vi "scecmd-list-to-json.vi"(11 "sce-cmd-list":cluster{"字符串":string, "数组 2":string[]}[](array[cluster])) -> (0 "LV Text":string, 3 "<JSON>":string caption="<JSON>Object")   [LabVIEW 2019]
uses:
  b78e4e2b-07cc-4402-99e5-c8c8689a2c4a.vi
  79eddf31-7dbf-49f6-a314-521278fd7013.vi
  3a01fc26-5e33-4aa7-adf9-b5ac6e867385.vi
  10d2d137-27d5-4f8a-8f99-ee01ed841b88.vi
  6bf9a7dc-aad9-4d5c-b2fa-1059882cb968.vi
  <vilib>/JDP Science/JSONtext/support/Format JSON Object.vi
  <vilib>/JDP Science/JSONtext/Variant to JSON Text.vi
  <vilib>/JDP Science/JSONtext/Get all Object Items.vi
  <vilib>/JDP Science/JSONtext/Set Multiple Object Items.vi
  <vilib>/JDP Science/JSONtext/JSONtext.lvlib
  <vilib>/addons/Tools/Unicode/UTF8 Tools.lvlib
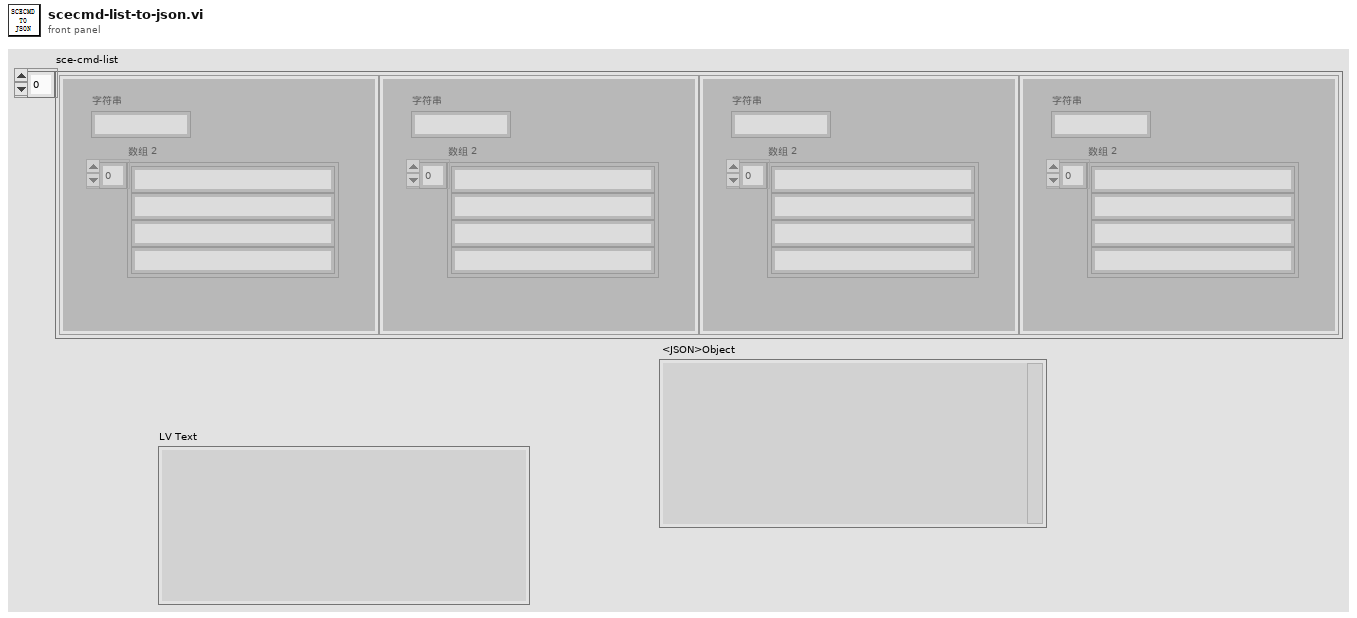
[diagram p1: front panel]
types:
  T1 = cluster{"场景":string, "open":cluster{"ID":dbl, "payload":string[]}, "close":cluster{"ID":dbl, "payload":string[]}, "common":cluster{"ID":dbl, "payload":string[]}}[]
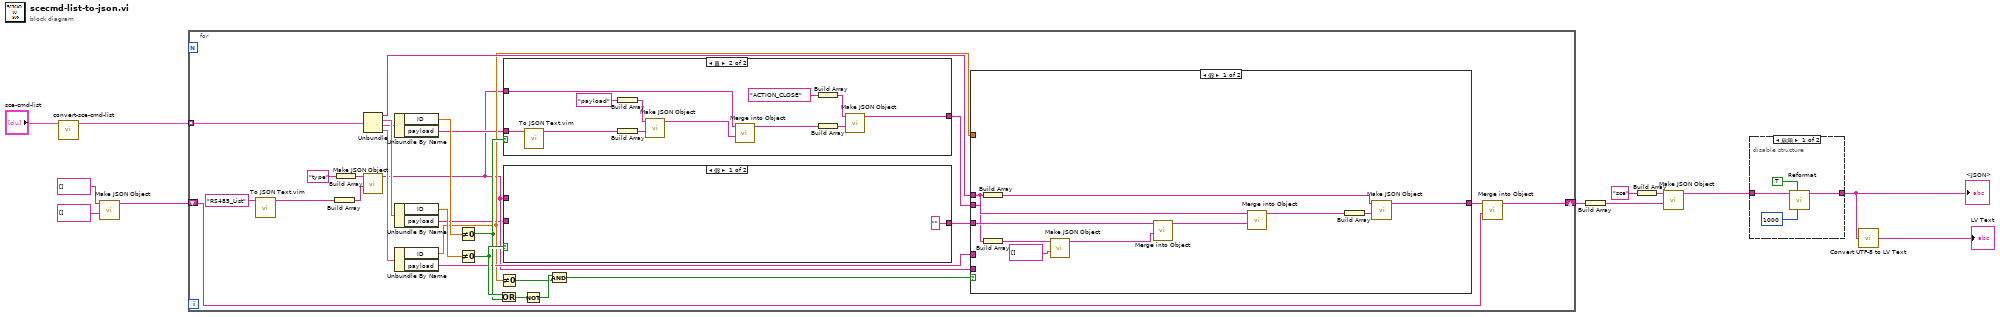
[diagram p0: block diagram]
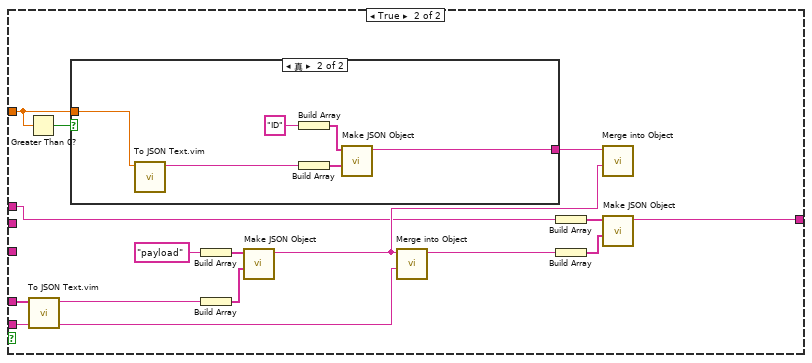
[diagram p3: hidden frame]
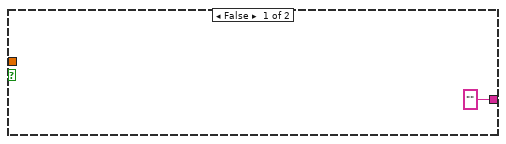
[diagram p4: hidden frame]
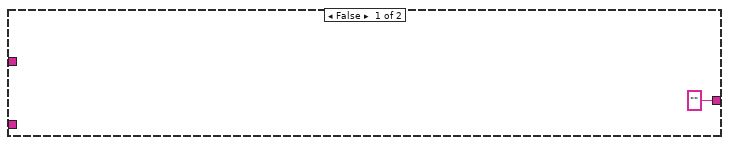
[diagram p5: hidden frame]
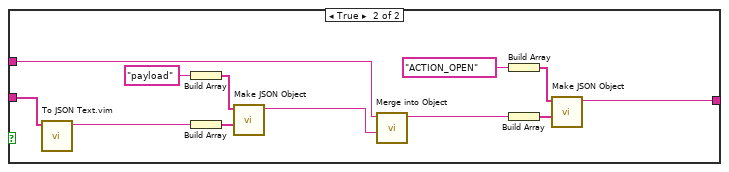
[diagram p6: hidden frame]
diagram:
  n1 = call "convert-sce-cmd-list.vi"("sce-cmd-list"="sce-cmd-list") -> ("场景-cmd-list"=w11:T1)  [unwired: 10 in]
  n2 = call <vilib>:"Make JSON Object.vi"("JSON Items"=string[] [], "Item Names"=string[] []) -> ("<JSON>"=w8:string)  [unwired: 8 in, 1 out]
  n3 = for {
    tunnel: w11 -> [w40] mode=indexing
    shift-right: [w14] -> w6
    shift-left: w8 -> [w13]
    n4 = call "To JSON Text.vim"("Anything"="RS485_List") -> ("<JSON>"=w26:string)  [unwired: 9 in, 1 out]
    n5 = Build Array(w26) -> (w25:string[])
    n6 = Build Array("type") -> (w27:string[])
    n7 = Unbundle(w40) -> ("场景"=w23:string, "open"=w39:cluster{"ID":dbl, "payload":string[]}, "close"=w38:cluster{"ID":dbl, "payload":string[]}, "common"=w37:cluster{"ID":dbl, "payload":string[]})
    n8 = call <vilib>:"Make JSON Object.vi"("JSON Items"=w25, "Item Names"=w27) -> ("<JSON>"=w19:string)  [unwired: 8 in, 1 out]
    n9 = Unbundle By Name(w38) -> ("ID"=w35:dbl, "payload"=w20:string[])
    n10 = Unbundle By Name(w39) -> ("ID"=w36:dbl, "payload"=w18:string[])
    n11 = Unbundle By Name(w37) -> ("ID"=w21:dbl, "payload"=w22:string[])
    n12 = Not Equal To 0?(x=w35) -> (x != 0?=w33:bool)
    n13 = Not Equal To 0?(x=w36) -> (x != 0?=w34:bool)
    n14 = Not Equal To 0?(x=w21) -> (x != 0?=w30:bool)
    n15 = Or(x=w34, y=w33) -> (x .or. y?=w32:bool)
    n16 = case shown="真" w33 {
      tunnel: w20 -> [_ w84]
      tunnel: w19 -> [_ w81]
      tunnel: ["" ("<JSON>") w75] -> w17
      frame False {
      }
      frame True {
        n17 = call "To JSON Text.vim"("Anything"=w84) -> ("<JSON>"=w83:string)  [unwired: 9 in, 1 out]
        n18 = Build Array("payload") -> (w85:string[])
        n19 = Build Array(w83) -> (w82:string[])
        n20 = call <vilib>:"Make JSON Object.vi"("JSON Items"=w82, "Item Names"=w85) -> ("<JSON>"=w80:string)  [unwired: 8 in, 1 out]
        n21 = call <vilib>:"Merge into Object.vi"("JSON Object to Merge"=w80, "JSON"=w81) -> ("<JSON>"=w76:string)  [unwired: 7 in, 1 out]
        n22 = Build Array("ACTION_CLOSE") -> (w79:string[])
        n23 = Build Array(w76) -> (w78:string[])
        n24 = call <vilib>:"Make JSON Object.vi"("JSON Items"=w78, "Item Names"=w79) -> ("<JSON>"=w75:string)  [unwired: 8 in, 1 out]
      }
    }
    n25 = case shown="假" w34 {
      tunnel: w19 -> [_ w94]
      tunnel: w18 -> [_ w93]
      tunnel: ["" ("<JSON>") w88] -> w16
      frame False {
      }
      frame True {
        n26 = call "To JSON Text.vim"("Anything"=w93) -> ("<JSON>"=w97:string)  [unwired: 9 in, 1 out]
        n27 = Build Array("payload") -> (w96:string[])
        n28 = Build Array(w97) -> (w98:string[])
        n29 = call <vilib>:"Make JSON Object.vi"("JSON Items"=w98, "Item Names"=w96) -> ("<JSON>"=w99:string)  [unwired: 8 in, 1 out]
        n30 = call <vilib>:"Merge into Object.vi"("JSON Object to Merge"=w99, "JSON"=w94) -> ("<JSON>"=w91:string)  [unwired: 7 in, 1 out]
        n31 = Build Array("ACTION_OPEN") -> (w89:string[])
        n32 = Build Array(w91) -> (w90:string[])
        n33 = call <vilib>:"Make JSON Object.vi"("JSON Items"=w90, "Item Names"=w89) -> ("<JSON>"=w88:string)  [unwired: 8 in, 1 out]
      }
    }
    n34 = Not(x=w32) -> (.not. x?=w31:bool)
    n35 = And(x=w31, y=w30) -> (x .and. y?=w29:bool)
    n36 = case shown="假" w29 {
      tunnel: w23 -> [w45 w56]
      tunnel: w22 -> [_ w59]
      tunnel: w21 -> [_ w66]
      tunnel: w19 -> [_ w57]
      tunnel: w17 -> [w48 _]
      tunnel: w16 -> [w50 _]
      tunnel: [w41 w52] -> w15
      frame False {
        n37 = Build Array(w45) -> (w44:string[])
        n38 = Build Array(w45) -> (w51:string[])
        n39 = call <vilib>:"Make JSON Object.vi"("JSON Items"=string[] [], "Item Names"=w51) -> ("<JSON>"=w49:string)  [unwired: 8 in, 1 out]
        n40 = call <vilib>:"Merge into Object.vi"("JSON Object to Merge"=w49, "JSON"=w50) -> ("<JSON>"=w47:string)  [unwired: 7 in, 1 out]
        n41 = call <vilib>:"Merge into Object.vi"("JSON Object to Merge"=w47, "JSON"=w48) -> ("<JSON>"=w43:string)  [unwired: 7 in, 1 out]
        n42 = Build Array(w43) -> (w42:string[])
        n43 = call <vilib>:"Make JSON Object.vi"("JSON Items"=w42, "Item Names"=w44) -> ("<JSON>"=w41:string)  [unwired: 8 in, 1 out]
      }
      frame True {
        n44 = Greater Than 0?(x=w66) -> (x > 0?=w65:bool)
        n45 = call "To JSON Text.vim"("Anything"=w59) -> ("<JSON>"=w62:string)  [unwired: 9 in, 1 out]
        n46 = case shown="真" w65 {
          tunnel: w66 -> [_ w69]
          tunnel: ["" ("<JSON>") w68] -> w60
          frame False {
          }
          frame True {
            n47 = call "To JSON Text.vim"("Anything"=w69) -> ("<JSON>"=w72:string)  [unwired: 9 in, 1 out]
            n48 = Build Array("ID") -> (w71:string[])
            n49 = Build Array(w72) -> (w73:string[])
            n50 = call <vilib>:"Make JSON Object.vi"("JSON Items"=w73, "Item Names"=w71) -> ("<JSON>"=w68:string)  [unwired: 8 in, 1 out]
          }
        }
        n51 = Build Array("payload") -> (w63:string[])
        n52 = Build Array(w62) -> (w61:string[])
        n53 = call <vilib>:"Make JSON Object.vi"("JSON Items"=w61, "Item Names"=w63) -> ("<JSON>"=w58:string)  [unwired: 8 in, 1 out]
        n54 = call <vilib>:"Merge into Object.vi"("JSON Object to Merge"=w57, "JSON"=w58) -> ("<JSON>"=w54:string)  [unwired: 7 in, 1 out]
        n55 = Build Array(w56) -> (w55:string[])
        n56 = Build Array(w54) -> (w53:string[])
        n57 = call <vilib>:"Merge into Object.vi"("JSON Object to Merge"=w58, "JSON"=w60) -> ()  [unwired: 7 in, 2 out]
        n58 = call <vilib>:"Make JSON Object.vi"("JSON Items"=w53, "Item Names"=w55) -> ("<JSON>"=w52:string)  [unwired: 8 in, 1 out]
      }
    }
    n59 = call <vilib>:"Merge into Object.vi"("JSON Object to Merge"=w13, "JSON"=w15) -> ("<JSON>"=w14:string)  [unwired: 7 in, 1 out]
  }
  n60 = Build Array(w6) -> (w5:string[])
  n61 = Build Array("sce") -> (w4:string[])
  n62 = call <vilib>:"Make JSON Object.vi"("JSON Items"=w5, "Item Names"=w4) -> ("<JSON>"=w2:string)  [unwired: 8 in, 1 out]
  n63 = disable-structure shown="启用" {
    disable-tunnel: w2 -> [w103 w104]
    disable-tunnel: [w102 w104] -> w1
    frame Enabled {
      n64 = call <vilib>:"Reformat.vi"("Pretty Print Levels"=1000, "Alphabetically Sort Objects"=TRUE, "JSON"=w103) -> ("<JSON>First JSON Value\n\n<JSON>"=w102:string)  [unwired: 5 in, 3 out]
    }
    frame Disabled {
    }
  }
  "<JSON>" <- w1
  n65 = call <vilib>:"Convert UTF-8 to LV Text.vi"("UTF-8 Text"=w1) -> ("LV Text"=→"LV Text":string)  [unwired: 13 in, 1 out]
